vi "Example.vi"(10 "Baud Rate":u32(ring)=57600 items=["75"=75, "110"=110, "134"=134, "150"=150, "300"=300, "600"=600, "1200"=1200, "1800"=1800, "2400"=2400, "4800"=4800, "7200"=7200, "9600"=9600, "14400"=14400, "19200"=19200, "28800"=28800, "38400"=38400, "56000"=56000, "57600"=57600, "115200"=115200, "128000"=128000, "230400"=230400], 11 "Comport":refnum<visa-resource-name>="COM20") -> (0 "error out":errorcluster)   [LabVIEW 2020]
doc: "Initializes the library with a serial comport as the transport method"
uses:
  Controls/UI-Digital Pins.ctl
  Controls/UI-Digital Pin.ctl
  Controls/UI-PWM Pins.ctl
  Controls/UI-PWM Pin.ctl
  Controls/UI-Analog Pins.ctl
  Controls/UI-Analog Pin.ctl
panel:
  out "Connected":bool
  out "Firmata Firmware Name":string
  out "Firmata Firmware Version":string
  in  "Stop":bool
  in  "Tab Control":T1(tab)
  in  "Connect":bool
  in  "Connection Details":enum32{"Serial Communication", "Page 2"}(tab)
  in  "Select Transport Mode":enum16{"Serial Communication Port"}(ring)
  in  "Array 2":T2 caption="Digital Lines                             Direction                                         ON/OFF                     Value" {"Pin Value" format="%.2f V"}
  in  "Analog Lines":T4 {"Pin Value" format="%#_g V"}
  in  "PWM / Servo Lines":T6 {"Value" min=0.0 max=10.0 scale=0.0..10.0}
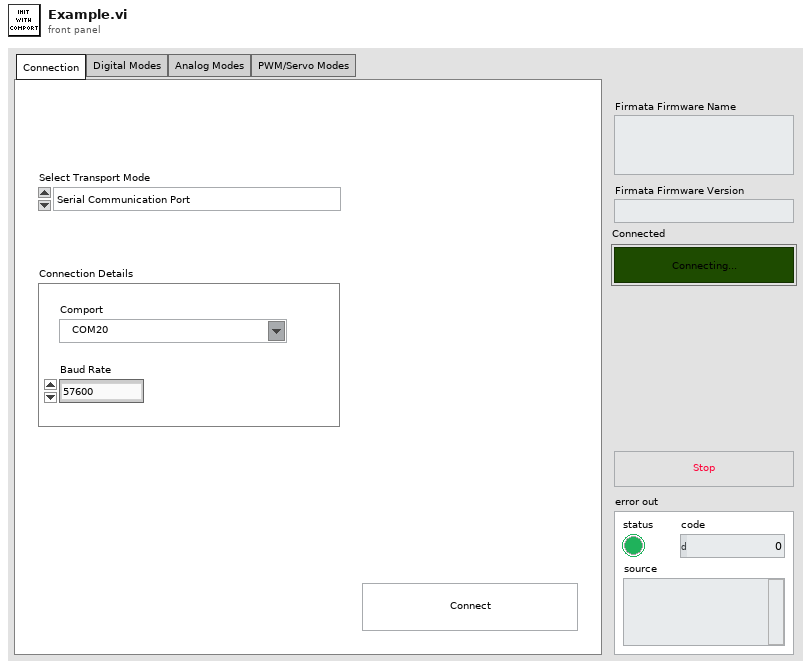
[diagram p1: front panel]
types:
  T1 = enum32{"Connection", "Digital Modes", "Analog Modes", "PWM/Servo Modes"}
  T2 = typedef "UI-Digital Pins.ctl" = T3[]
  T3 = typedef "UI-Digital Pin.ctl" = cluster{"IO Direction":u16, "Pin Direction":string, "DO Value":u16, "Pin Value":dbl, "Pin Index":string, "Pin Mode":string}
  T4 = typedef "UI-Analog Pins.ctl" = T5[]
  T5 = typedef "UI-Analog Pin.ctl" = cluster{"IO Direction":u16, "Pin Direction":string, "Pin Value":dbl, "Pin Index":string, "Pin Mode":string}
  T6 = typedef "UI-PWM Pins.ctl" = T7[]
  T7 = typedef "UI-PWM Pin.ctl" = cluster{"Pin Mode":u16, "Pin Mode":string, "Value":dbl, "Pin Index":string, "Pin Modes":string}
  T8 = enum16{"DigitalInput", "DigitalOutput", "AnalogInput", "PWM", "Servo", "Shift", "I2C", "OneWire", "Stepper", "Encoder", "Serial", "InputPullup", "Extended.SPI", "Extended.Sonar", "Extended.Tone", "Extended.DHT"}
  T9 = set{enum16{"DigitalInput", "DigitalOutput", "AnalogInput", "PWM", "Servo", "Shift", "I2C", "OneWire", "Stepper", "Encoder", "Serial", "InputPullup", "Extended.SPI", "Extended.Sonar", "Extended.Tone", "Extended.DHT"}}
  T10 = map{i32, cluster{"Supported Modes":cluster{"PinMode":enum16{"DigitalInput", "DigitalOutput", "AnalogInput", "PWM", "Servo", "Shift", "I2C", "OneWire", "Stepper", "Encoder", "Serial", "InputPullup", "Extended.SPI", "Extended.Sonar", "Extended.Tone", "Extended.DHT"}, "Resolution":u8}[], "Analog Channel":u8, "Pin Name":string}}
  T11 = cluster{"Supported Modes":cluster{"PinMode":enum16{"DigitalInput", "DigitalOutput", "AnalogInput", "PWM", "Servo", "Shift", "I2C", "OneWire", "Stepper", "Encoder", "Serial", "InputPullup", "Extended.SPI", "Extended.Sonar", "Extended.Tone", "Extended.DHT"}, "Resolution":u8}[], "Analog Channel":u8, "Pin Name":string}
  T12 = cluster{"PinMode":enum16{"DigitalInput", "DigitalOutput", "AnalogInput", "PWM", "Servo", "Shift", "I2C", "OneWire", "Stepper", "Encoder", "Serial", "InputPullup", "Extended.SPI", "Extended.Sonar", "Extended.Tone", "Extended.DHT"}, "Resolution":u8}[]
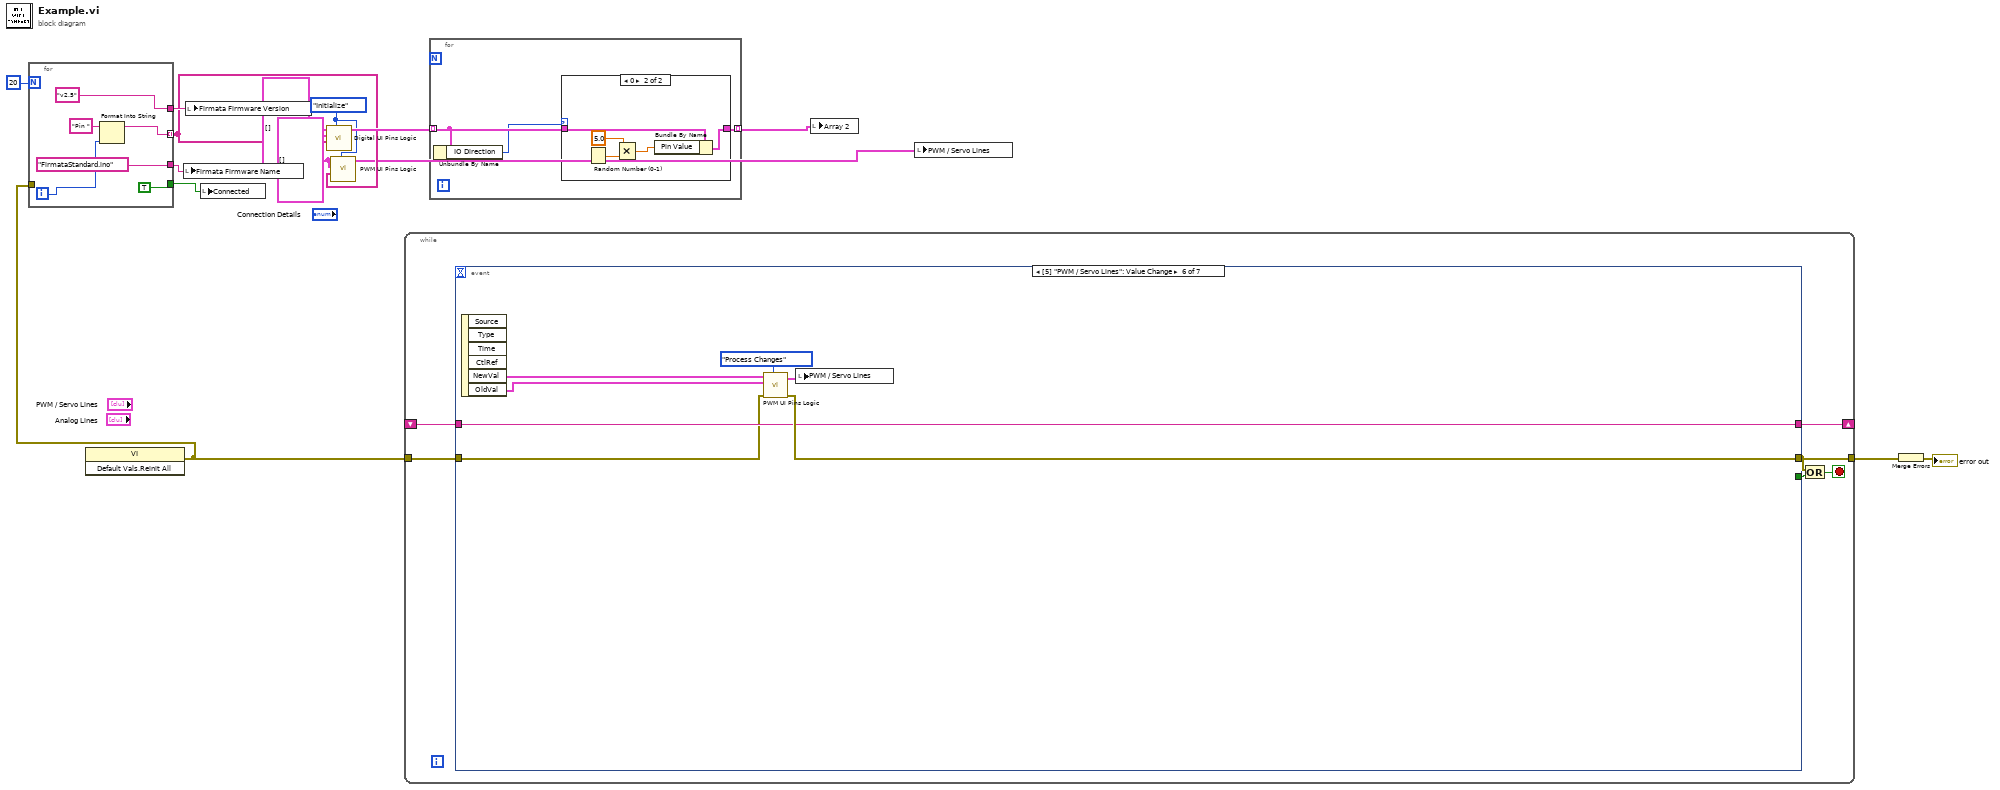
[diagram p0: block diagram]
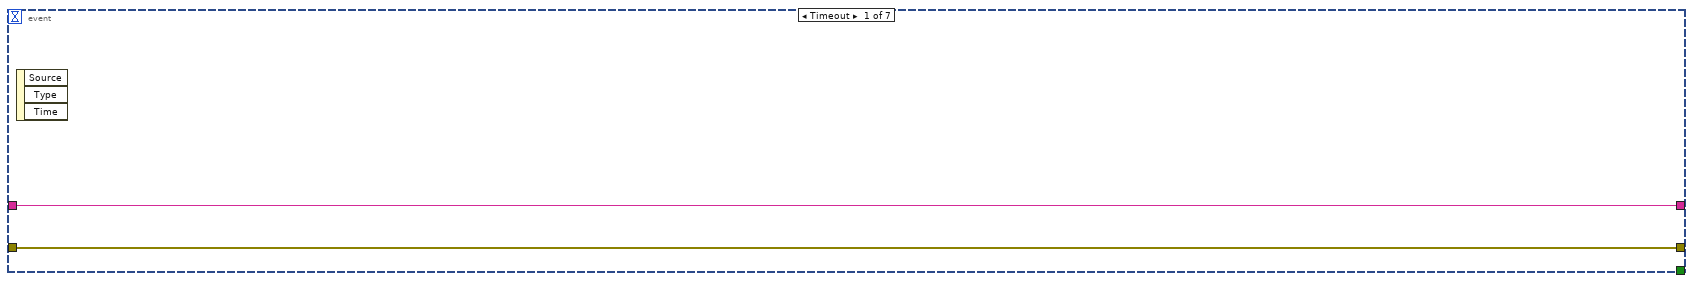
[diagram p3: hidden frame]
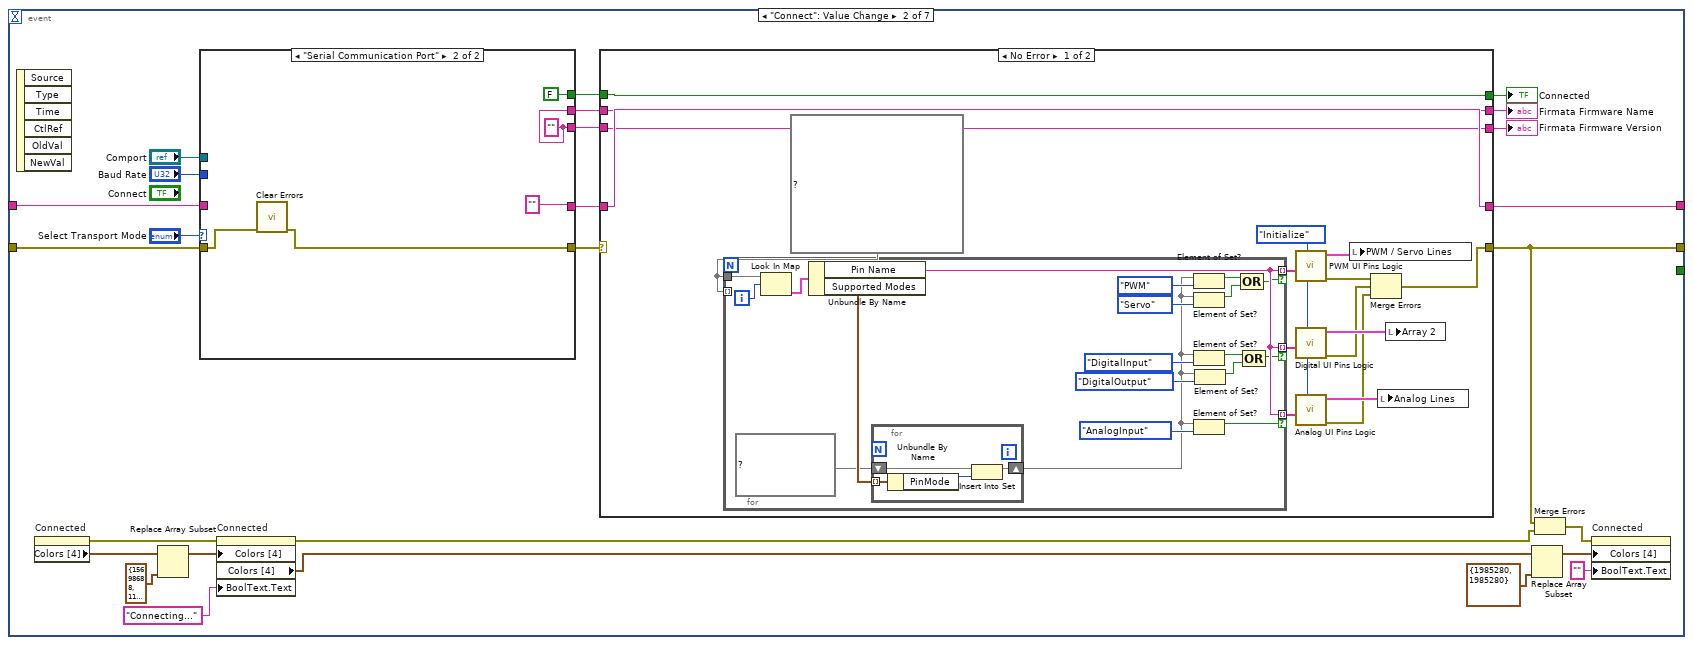
[diagram p4: hidden frame]
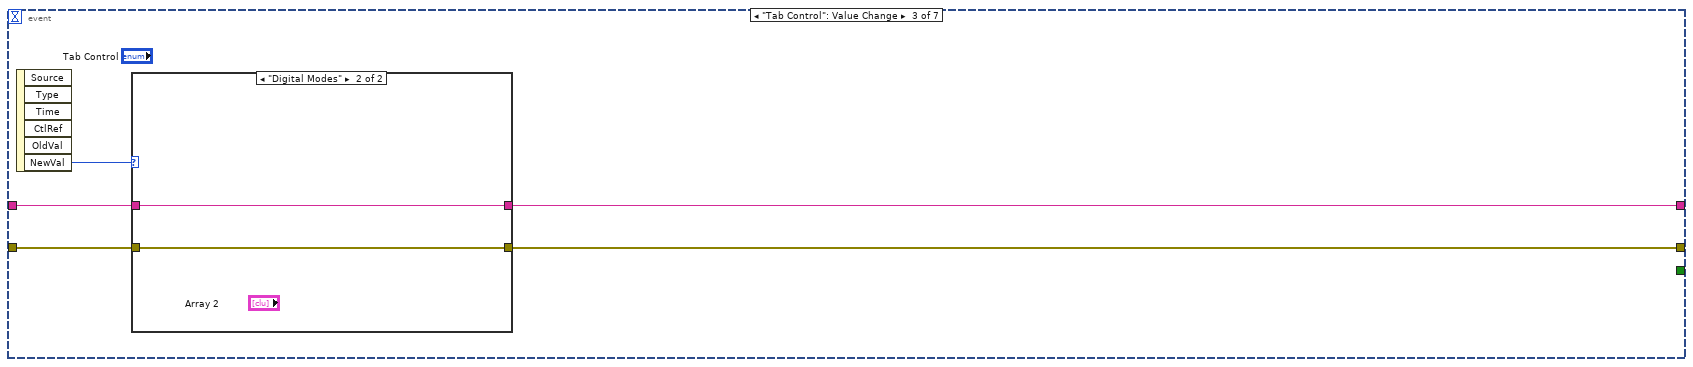
[diagram p7: hidden frame]
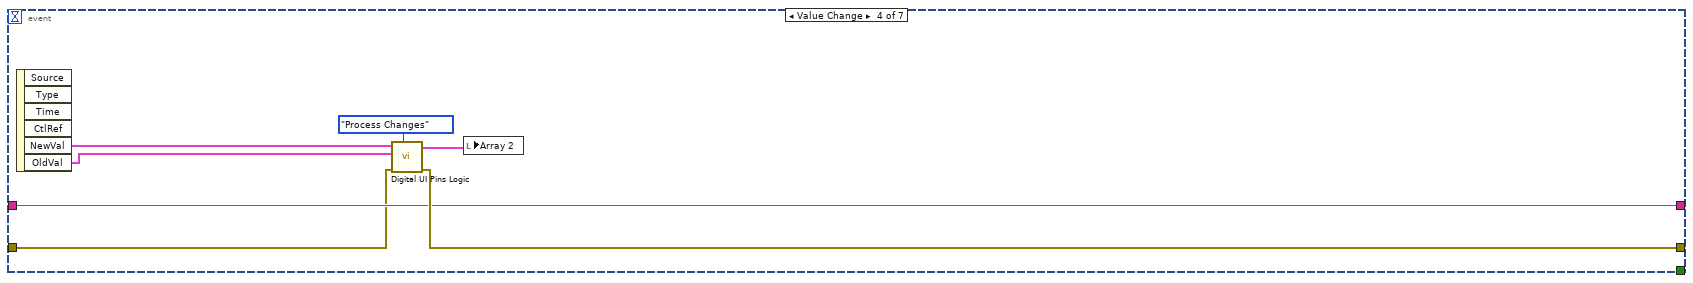
[diagram p9: hidden frame]
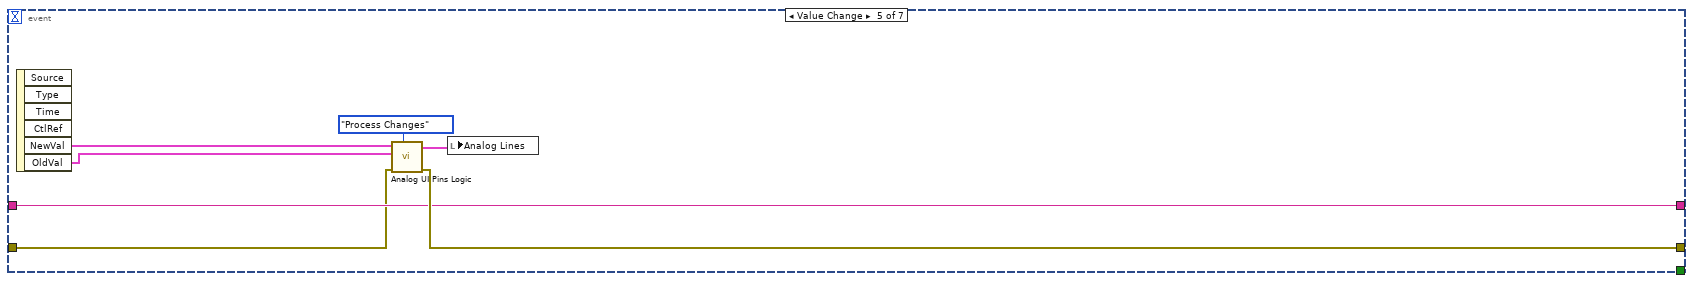
[diagram p10: hidden frame]
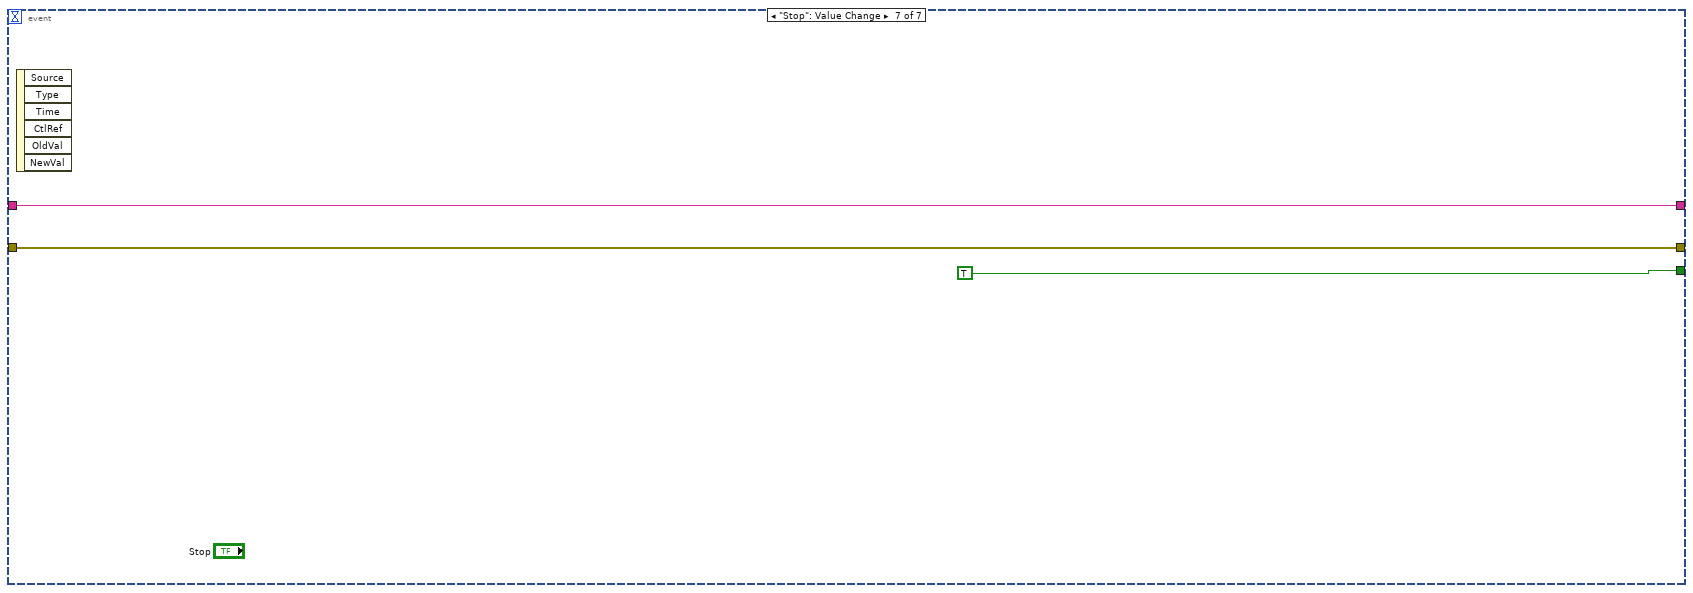
[diagram p11: hidden frame]
diagram:
  w3 = T6 [] ("NewVal")
  w12 = T2 [] ("NewVal")
  w4 = enum16{"Initialize", "Process Changes"}."Initialize" ("Mode")
  n1 = invoke class="VI" method="Default Vals.Reinit All"() -> (error out=w10:errorcluster)  [unwired: 3 in, 2 out]
  n2 = for {
    N: 20 -> [_]
    tunnel: [w19] -> w2 mode=indexing
    tunnel: w10 -> [_]
    tunnel: ["FirmataStandard.ino"] -> w9
    tunnel: [TRUE] -> w8
    tunnel: ["v2.5"] -> w7
    i -> [w20]
    n3 = Format Into String(initial string="Pin ", w20) -> (resulting string=w19:string)  [unwired: 2 in, 1 out]
  }
  n4 = local write "Firmata Firmware Name"(w9) -> ()
  n5 = local write "Firmata Firmware Version"(w7) -> ()
  n6 = local write "Connected"(w8) -> ()
  n7 = call "Digital UI Pins Logic.vi"("Mode"=w4, "Initial Pin Names"=w2, "OldVal"=w12, "NewVal"=w12) -> ("Updated Value"=w5:T2)  [unwired: 6 in, 1 out]
  n8 = call "PWM UI Pins Logic.vi"("Mode"=w4, "Initial Pin Names"=w2, "OldVal"=w3, "NewVal"=w3) -> ("Updated Value"=w1:T6)  [unwired: 6 in, 1 out]
  n9 = while {
    shift-right: [w26] -> _
    shift-left: _ -> [w25]
    tunnel: w10 -> [w24]
    tunnel: [w23] -> w13
    stop <- w21 stop-if-true
    n10 = event shown="[5] \"PWM / Servo Lines\": Value Change" {
      selector: _ -> [_ _ _ _ _ _ _]
      dyn-events: _ -> [_ _ _ _ _ _ _]
      timeout: _ -> [_ _ _ _ _ _ _]
      tunnel: [_ _ _ _ _ _ TRUE] -> w22
      tunnel: [w28 w47 w108 w117 w124 w131 w138] -> w26
      tunnel: w25 -> [w28 w52 w107 w117 w124 w131 w138]
      tunnel: [w27 w32 w110 w118 w125 w132 w137] -> w23
      tunnel: w24 -> [w27 w54 w109 w116 w123 w130 w137]
      event Timeout {
        n11 = event-data() -> ()  [unwired: 1 in, 3 out]
      }
      event "Connect": Value Change {
        n12 = event-data() -> ()  [unwired: 1 in, 6 out]
        n13 = property on="Connected" class="Bool (strict)"() -> (error out=w36:errorcluster, "Colors [4]"=w38:cluster{u32, u32}[])  [unwired: 2 in, 1 out]
        n14 = Replace Array Subset(array=w38, new element=cluster{u32, u32} {15698688, 11820800} ("new element/subarray")) -> (w35:cluster{u32, u32}[])  [unwired: 1 in]
        n15 = case shown="\"Serial Communication Port\"" "Select Transport Mode" {
          tunnel: w54 -> [w99 w104]
          tunnel: [w100 ""] -> w48
          tunnel: [w99 w105] -> w49
          tunnel: w52 -> [w100 _]
          tunnel: "Baud Rate" -> [_ _]
          tunnel: "Comport" -> [_ _]
          tunnel: [_ FALSE ("Connected")] -> w46
          tunnel: [_ w103] -> w45
          tunnel: [_ w103] -> w44
          frame Default {
          }
          frame "Serial Communication Port" {
            w103 = "" ("FirmataFirmwareVersion")
            n16 = call <vilib>:"Clear Errors.vi"("error in (no error)"=w104) -> ("error out"=w105:errorcluster)  [unwired: 5 in, 1 out]
          }
        }
        n17 = property on="Connected" class="Bool (strict)"(error in=w36, "Colors [4]"=w35, "BoolText.Text"="Connecting..." ("Boolean Text.Text")) -> (error out=w31:errorcluster, "Colors [4]"=w33:cluster{u32, u32}[])  [unwired: 1 in, 1 out]
        n18 = case shown="No Error" w49 {
          selector: w49 -> [_ w98]
          tunnel: [w65 w98] -> w32
          tunnel: [w70 w97] -> w47
          tunnel: w48 -> [w70 w97]
          tunnel: w46 -> [w64 w94]
          tunnel: w45 -> [w62 w96]
          tunnel: w44 -> [w63 w95]
          tunnel: [w64 w94] -> w43
          tunnel: [w63 w95] -> w42
          tunnel: [w62 w96] -> w41
          frame No Error {
            w55 = T10 {} ("Board Capabilities")
            w60 = enum16{"Initialize", "Process Changes"}."Initialize" ("Mode")
            n19 = for {
              tunnel: w55 -> [w89]
              tunnel: w55 -> [_] mode=indexing
              tunnel: [w84] -> w58 mode=indexing if=w73
              tunnel: [w84] -> w57 mode=indexing if=w72
              tunnel: [w84] -> w56 mode=indexing if=w71
              i -> [w88]
              n20 = Look In Map(map=w89, key=w88) -> (value=w87:T11)  [unwired: 1 in, 1 out]
              n21 = Unbundle By Name(w87) -> ("Pin Name"=w84:string, "Supported Modes"=w86:T12)
              n22 = for {
                tunnel: w86 -> [w93] mode=indexing
                shift-right: [w90] -> w76
                shift-left: T9 {} ("set in") -> [w91]
                n23 = Unbundle By Name(w93) -> ("PinMode"=w92:T8)
                n24 = Insert Into Set(10:w92, 11:w91) -> (3:w90:T9)  [unwired: 1 out]
              }
              n25 = Element of Set?(10:T8."PWM" ("element"), 11:w76) -> (3:w74:bool)
              n26 = Element of Set?(10:T8."Servo" ("element"), 11:w76) -> (3:w75:bool)
              n27 = Element of Set?(10:T8."DigitalInput" ("element"), 11:w76) -> (3:w78:bool)
              n28 = Element of Set?(10:T8."AnalogInput" ("element"), 11:w76) -> (3:w71:bool)
              n29 = Element of Set?(10:T8."DigitalOutput" ("element"), 11:w76) -> (3:w79:bool)
              n30 = Compound Arithmetic op=OR(w74, w75) -> (w73:bool)
              n31 = Compound Arithmetic op=OR(w78, w79) -> (w72:bool)
            }
            n32 = call "PWM UI Pins Logic.vi"("Mode"=w60, "Initial Pin Names"=w58) -> ("error out"=w67:errorcluster, "Updated Value"=w69:T6)  [unwired: 8 in]
            n33 = call "Digital UI Pins Logic.vi"("Mode"=w60, "Initial Pin Names"=w57) -> ("error out"=w66:errorcluster, "Updated Value"=w68:T2)  [unwired: 8 in]
            n34 = call "Analog UI Pins Logic.vi"("Mode"=w60, "Initial Pin Names"=w56) -> ("error out"=w59:errorcluster, "Updated Value"=w61:T4)  [unwired: 8 in]
            n35 = local write "PWM / Servo Lines"(w69) -> ()
            n36 = Merge Errors(w67, w66, w59) -> (w65:errorcluster)
            n37 = local write "Analog Lines"(w61) -> ()
            n38 = local write "Array 2"(w68) -> ()
          }
          frame Error {
          }
        }
        "Firmata Firmware Name" <- w42
        "Firmata Firmware Version" <- w41
        "Connected" <- w43
        n39 = Replace Array Subset(array=w33, new element=cluster{"Numeric":u32, "Numeric":u32} {"Numeric"=1985280, "Numeric"=1985280} ("element")) -> (w40:cluster{u32, u32}[])  [unwired: 1 in]
        n40 = Merge Errors(w32, w31) -> (w30:errorcluster)
        n41 = property on="Connected" class="Bool (strict)"(error in=w30, "Colors [4]"=w40, "BoolText.Text"="" ("Boolean Text.Text")) -> ()  [unwired: 1 in, 2 out]
      }
      event "Tab Control": Value Change {
        n42 = event-data() -> ("NewVal"=w106:T1)  [unwired: 1 in, 5 out]
        n43 = case shown="\"Digital Modes\"" w106 {
          tunnel: [w112 w114] -> w110
          tunnel: w109 -> [w112 w114]
          tunnel: [w111 w113] -> w108
          tunnel: w107 -> [w111 w113]
          frame "Connection", Default {
          }
          frame "Digital Modes" {
          }
        }
      }
      event Value Change {
        n44 = event-data() -> ("NewVal"=w121:T2, "OldVal"=w120:T2)  [unwired: 1 in, 4 out]
        n45 = call "Digital UI Pins Logic.vi"("Mode"=enum16{"Initialize", "Process Changes"}."Process Changes", "error in"=w116, "OldVal"=w120, "NewVal"=w121) -> ("error out"=w118:errorcluster, "Updated Value"=w119:T2)  [unwired: 6 in]
        n46 = local write "Array 2"(w119) -> ()
      }
      event Value Change {
        n47 = event-data() -> ("NewVal"=w128:T4, "OldVal"=w127:T4)  [unwired: 1 in, 4 out]
        n48 = call "Analog UI Pins Logic.vi"("Mode"=enum16{"Initialize", "Process Changes"}."Process Changes", "error in"=w123, "OldVal"=w127, "NewVal"=w128) -> ("error out"=w125:errorcluster, "Updated Value"=w126:T4)  [unwired: 6 in]
        n49 = local write "Analog Lines"(w126) -> ()
      }
      event Value Change {
        n50 = event-data() -> ("NewVal"=w135:T6, "OldVal"=w134:T6)  [unwired: 1 in, 4 out]
        n51 = call "PWM UI Pins Logic.vi"("Mode"=enum16{"Initialize", "Process Changes"}."Process Changes", "error in"=w130, "OldVal"=w134, "NewVal"=w135) -> ("error out"=w132:errorcluster, "Updated Value"=w133:T6)  [unwired: 6 in]
        n52 = local write "PWM / Servo Lines"(w133) -> ()
      }
      event "Stop": Value Change {
        n53 = event-data() -> ()  [unwired: 1 in, 6 out]
      }
    }
    n54 = Compound Arithmetic op=OR(w23, w22) -> (w21:bool)
  }
  n55 = for {
    tunnel: [w141] -> w6 mode=indexing
    tunnel: w5 -> [w140] mode=indexing
    n56 = Unbundle By Name(w140) -> ("IO Direction"=w139:u16)
    n57 = case shown="0" w139 {
      tunnel: [w142 w147] -> w141
      tunnel: w140 -> [w142 w146]
      frame Default {
      }
      frame 0 {
        n58 = Random Number (0-1)() -> (number: 0 to 1=w145:dbl)
        n59 = Multiply(x=5.0, y=w145) -> (x*y=w143:dbl)
        n60 = Bundle By Name(cluster=w146, "Pin Value"=w143) -> (w147:T3)
      }
    }
  }
  n61 = local write "Array 2"(w6) -> ()
  n62 = local write "PWM / Servo Lines"(w1) -> ()
  n63 = Merge Errors(w13) -> (→"error out":errorcluster)
